vi "Timer_kernel.vi"(8 "Error In":errorcluster, 10 "Timer Inputs":T2, 11 "Timer States":T3) -> (0 "Error Out":errorcluster, 2 "Timer Outputs":T1, 3 "Timer States out":T3)   [LabVIEW 2013]
doc: "This is the kernel of the functional global variable (FGV) that acts as a timer for the SVM burner test VI. It\naccepts a target time and status Booleans as arguments, and returns status Booleans and elapsed time\nindicating whether the flame has been relit, has been lit for long enough, or has blown out.\nArgs:\n Target time (float): target time in seconds for the VI to wait before accepting a flame as stable\n relight? (bool): indicates when we are relighting the flame (do not indicate that flame has blown out)\n flame? (bool): indicates when a flame is detected and the timer should count\n\nStates:\n Elapsed time (float): time in seconds that the timer has been running and detecting a flame\n Previous timestamp (float): time stamp the last time the timer updated. Used to update elapsed time.\n\nReturns:\n target reached? (bool): indicates when the flame has been lit for the target duration.\n flame out? (bool): indicates when the flame has blown out. Will not turn True unless relight? is False.\n flame lit? (bool): indicates when the flame has been lit. Will not turn True unless relight? is True."
uses:
  Controls/timer_state_cluster.ctl
  Controls/timer_input_cluster.ctl
  Controls/timer_output_cluster.ctl
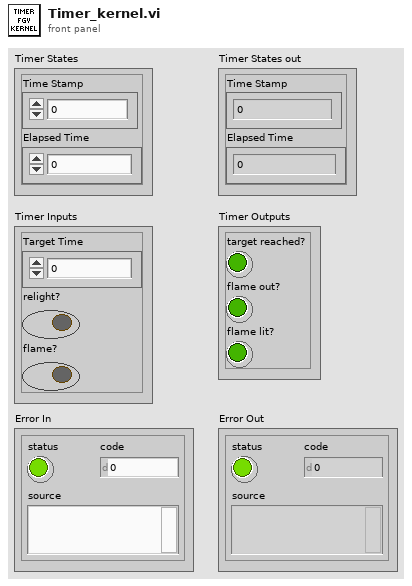
[diagram p1: front panel]
types:
  T1 = typedef "timer_output_cluster.ctl" = cluster{"target reached?":bool, "flame out?":bool, "flame lit?":bool}
  T2 = typedef "timer_input_cluster.ctl" = cluster{"Target Time":dbl, "relight?":bool, "flame?":bool}
  T3 = typedef "timer_state_cluster.ctl" = cluster{"Time Stamp":dbl, "Elapsed Time":dbl}
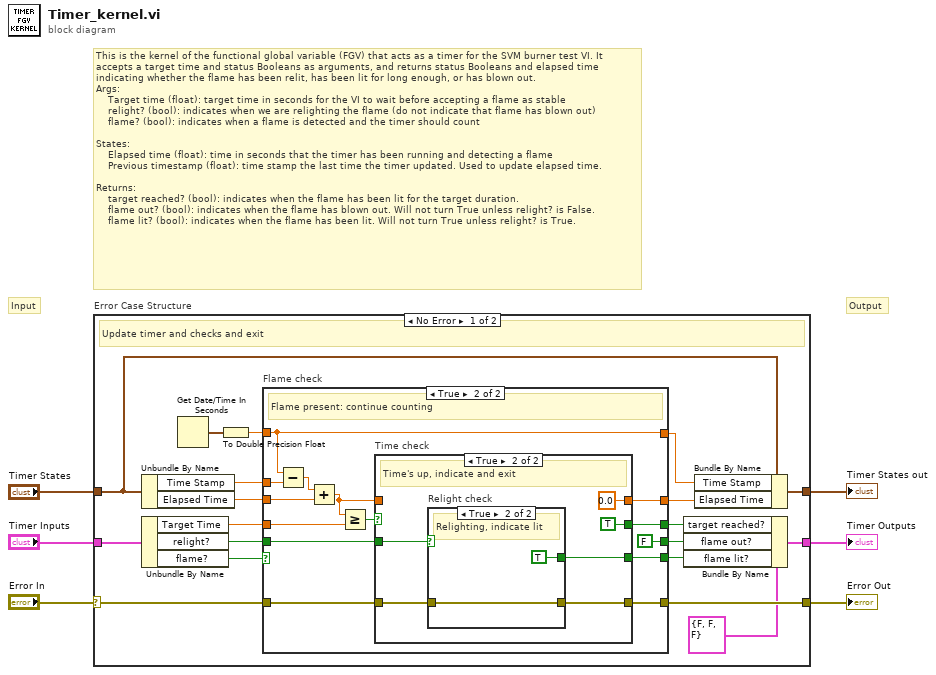
[diagram p0: block diagram]
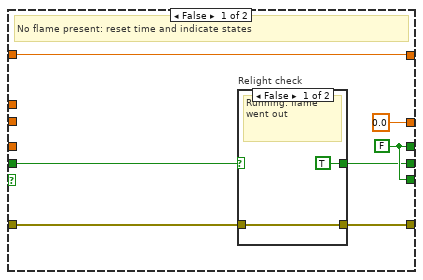
[diagram p2: hidden frame]
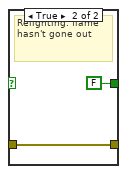
[diagram p3: hidden frame]
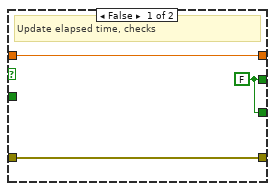
[diagram p4: hidden frame]
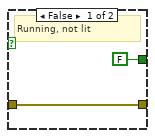
[diagram p5: hidden frame]
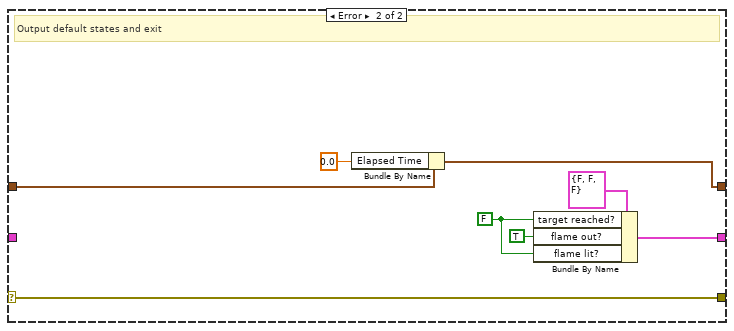
[diagram p6: hidden frame]
diagram:
  # "Output"
  # "Input"
  # "This is the kernel of the functional global variable (FGV) that acts as a timer for the SVM burner test VI. It\naccepts a target time and status Booleans as arguments, and returns status Booleans and elapsed time\nindicating whether the flame has been relit, has been lit for long enough, or has blown out.\nArgs:\n    Target time (float): target time in seconds for the VI to wait before accepting a flame as stable\n    relight? (bool): indicates when we are relighting the flame (do not indicate that flame has blown out)\n    flame? (bool): indicates when a flame is detected and the timer should count\n\nStates:\n    Elapsed time (float): time in seconds that the timer has been running and detecting a flame\n    Previous timestamp (float): time stamp the last time the timer updated. Used to update elapsed time.\n\nReturns:\n    target reached? (bool): indicates when the flame has been lit for the target duration.\n    flame out? (bool): indicates when the flame has blown out. Will not turn True unless relight? is False.\n    flame lit? (bool): indicates when the flame has been lit. Will not turn True unless relight? is True."
  n1 = case "Error Case Structure" shown="No Error" "Error In" {
    selector: "Error In" -> [w22 w71]
    tunnel: [w21 w71] -> w5
    tunnel: "Timer States" -> [w20 w70]
    tunnel: [w19 w68] -> w3
    tunnel: "Timer Inputs" -> [w15 _]
    tunnel: [w9 w64] -> w1
    frame No Error {
      # "Update timer and checks and exit"
      n2 = Unbundle By Name(w20) -> ("Time Stamp"=w24:dbl, "Elapsed Time"=w23:dbl)
      n3 = Unbundle By Name(w15) -> ("Target Time"=w14:dbl, "relight?"=w13:bool, "flame?"=w12:bool)
      n4 = Get Date/Time In Seconds() -> (seconds since 1Jan1904=w25:timestamp)
      n5 = To Double Precision Float(number=w25) -> (double precision float=w18:dbl)
      n6 = case "Flame check" shown="True" w12 {
        tunnel: w18 -> [w32 w47]
        tunnel: w24 -> [_ w50]
        tunnel: w13 -> [w29 w41]
        tunnel: w14 -> [_ w46]
        tunnel: w23 -> [_ w48]
        tunnel: w22 -> [w28 w45]
        tunnel: [w27 w38] -> w21
        tunnel: [w32 w47] -> w17
        tunnel: [0.0 w43] -> w16
        tunnel: [w30 w40] -> w10
        tunnel: [w30 w39] -> w7
        tunnel: [w26 FALSE] -> w8
        frame False {
          w30 = FALSE
          # "No flame present: reset time and indicate states"
          n7 = case "Relight check" shown="False" w29 {
            tunnel: w28 -> [w34 w35]
            tunnel: [w34 w35] -> w27
            tunnel: [TRUE FALSE] -> w26
            frame False {
              # "Running: flame went out"
            }
            frame True {
              # "Relighting: flame hasn't gone out"
            }
          }
        }
        frame True {
          # "Flame present: continue counting"
          n8 = Subtract(x=w47, y=w50) -> (x-y=w49:dbl)
          n9 = Add(x=w49, y=w48) -> (x+y=w37:dbl)
          n10 = Greater Or Equal?(x=w37, y=w46) -> (x >= y?=w44:bool)
          n11 = case "Time check" shown="True" w44 {
            tunnel: w45 -> [w51 w58]
            tunnel: [w53 0.0] -> w43
            tunnel: w41 -> [_ w57]
            tunnel: [w52 TRUE] -> w40
            tunnel: [w52 w55] -> w39
            tunnel: [w51 w54] -> w38
            tunnel: w37 -> [w53 _]
            frame False {
              w52 = FALSE
              # "Update elapsed time, checks"
            }
            frame True {
              # "Time's up, indicate and exit"
              n12 = case "Relight check" shown="True" w57 {
                tunnel: w58 -> [w60 w62]
                tunnel: [FALSE TRUE] -> w55
                tunnel: [w60 w62] -> w54
                frame False {
                  # "Running, not lit"
                }
                frame True {
                  # "Relighting, indicate lit"
                }
              }
            }
          }
        }
      }
      n13 = Bundle By Name(cluster=T1 {"target reached?"=FALSE, "flame out?"=FALSE, "flame lit?"=FALSE} ("Timer Outputs 2"), "target reached?"=w10, "flame out?"=w8, "flame lit?"=w7) -> (w9:T1)
      n14 = Bundle By Name(cluster=w20, "Time Stamp"=w17, "Elapsed Time"=w16) -> (w19:T3)
    }
    frame Error {
      w65 = FALSE ("target reached?")
      # "Output default states and exit"
      n15 = Bundle By Name(cluster=w70, "Elapsed Time"=0.0) -> (w68:T3)
      n16 = Bundle By Name(cluster=T1 {"target reached?"=FALSE, "flame out?"=FALSE, "flame lit?"=FALSE} ("Timer Outputs 2"), "target reached?"=w65, "flame out?"=TRUE, "flame lit?"=w65) -> (w64:T1)
    }
  }
  "Error Out" <- w5
  "Timer States out" <- w3
  "Timer Outputs" <- w1
